vi "SettingsData.vi"(9 "Write (T)/Read (F)":bool, 11 "Settings in":T1) -> (3 "Settings out":T1)   [LabVIEW 2020]
uses:
  controls/PlayerSettings.ctl
  controls/PlayerMode.ctl
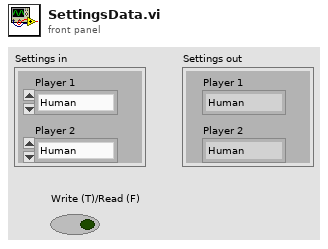
[diagram p1: front panel]
types:
  T1 = typedef "PlayerSettings.ctl" = cluster{"Player 1":T2, "Player 2":T2}
  T2 = typedef "PlayerMode.ctl" = enum16{"Human", "Bot Random", "Bot Intermidiate", "Bot Perfect Play"}
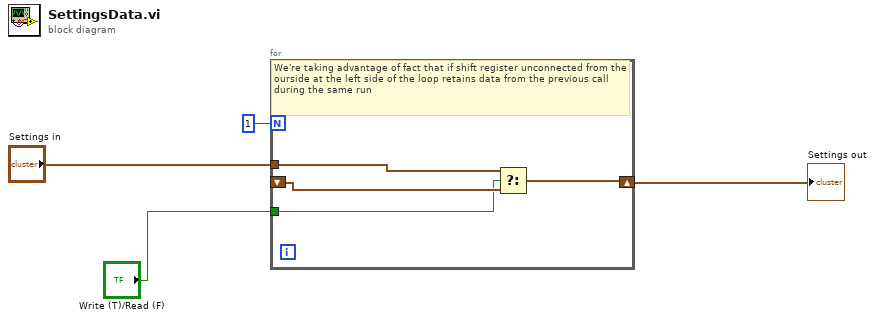
[diagram p0: block diagram]
diagram:
  n1 = for {
    N: 1 -> [_]
    shift-right: [w7] -> w4
    shift-left: _ -> [w6]
    tunnel: "Write (T)/Read (F)" -> [w5]
    tunnel: "Settings in" -> [w8]
    # "We're taking advantage of fact that if shift register unconnected from the ourside at the left side of the loop retains data from the previous call during the same run"
    n2 = Select(t=w8, s=w5, f=w6) -> (s? t:f=w7:T1)
  }
  "Settings out" <- w4
